vi "FPGA_CounterEncoderSourceConvertionLVSourceTypeToFPGAType.vi"(8 "error in (no error)":errorcluster, 11 "DigitalSource":T1={"DevStatus"={"status"=FALSE, "code"=0, "source"=""}, "AnalogTriggerMode?"=FALSE, "DigitalMode"={"DIO Channel"=enum."DIO 1"}, "AnalogTriggerMode"={"AnalogTriggerIndex"=enum."Trig 0", "OutputType"=enum."InWindow"}}) -> (0 "error out":errorcluster, 3 "FPGASource":T5={"Channel"=2.0, "Module"=0.0, "AnalogTrigger"=FALSE})   [LabVIEW 2017]
uses:
  <vilib>/Rock Robotics/SystemInterfaces/CounterEncoderSourceConvertion/FPGA_CounterEncoderSourceConvertionLVSourceType.ctl
  <vilib>/Rock Robotics/SystemInterfaces/DIO/FPGA_DIODigitalSourceChannel.ctl
  <vilib>/Rock Robotics/SystemInterfaces/AnalogTrigger/FPGA_AnalogTriggerIndex.ctl
  <vilib>/Rock Robotics/SystemInterfaces/AnalogTrigger/FPGA_AnalogTriggerOutType.ctl
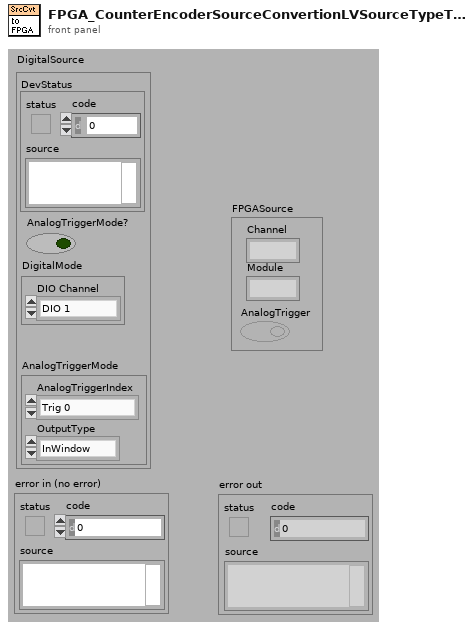
[diagram p1: front panel]
types:
  T1 = typedef "FPGA_CounterEncoderSourceConvertionLVSourceType.ctl" = cluster{"DevStatus":errorcluster, "AnalogTriggerMode?":bool, "DigitalMode":cluster{"DIO Channel":T2}, "AnalogTriggerMode":cluster{"AnalogTriggerIndex":T3, "OutputType":T4}}
  T2 = typedef "FPGA_DIODigitalSourceChannel.ctl" = enum8{"DIO 0", "DIO 1", "DIO 2", "DIO 3", "DIO 4", "DIO 5", "DIO 6", "DIO 7", "DIO 8", "DIO 9", "DIO MXP 0", "DIO MXP 1", "DIO MXP 2", "DIO MXP 3", "DIO MXP 4", "DIO MXP 5", "DIO MXP 6", "DIO MXP 7", "DIO MXP 8", "DIO MXP 9", "DIO MXP 10", "DIO MXP 11", "DIO MXP 12", "DIO MXP 13", "DIO MXP 14", "DIO MXP 15", "Disabled"}
  T3 = typedef "FPGA_AnalogTriggerIndex.ctl" = enum8{"Trig 0", "Trig 1", "Trig 2", "Trig 3", "Trig 4", "Trig 5", "Trig 6", "Trig 7", "Invalid"}
  T4 = typedef "FPGA_AnalogTriggerOutType.ctl" = enum16{"InWindow", "TriggerState", "Rising", "Falling"}
  T5 = cluster{"Channel":fxp<+,4,4>, "Module":fxp<+,1,1>, "AnalogTrigger":bool}
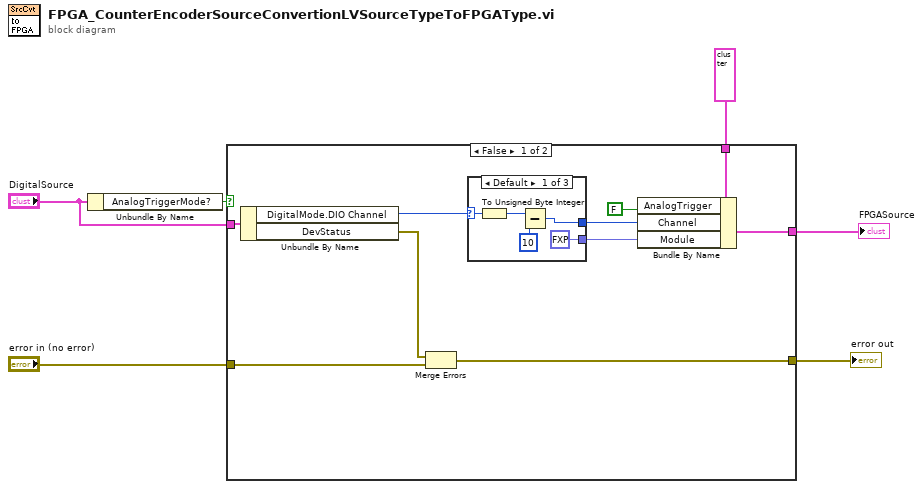
[diagram p0: block diagram]
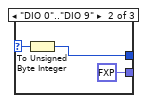
[diagram p2: hidden frame]
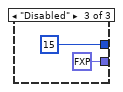
[diagram p3: hidden frame]
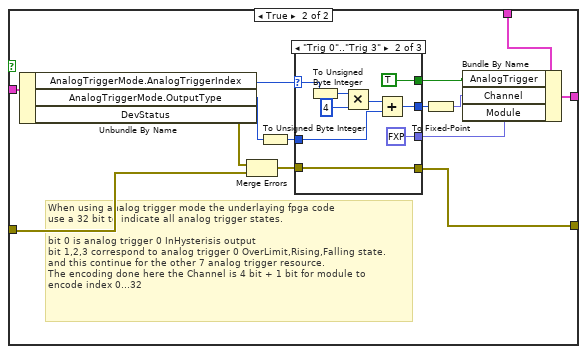
[diagram p4: hidden frame]
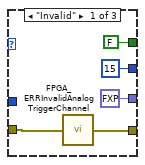
[diagram p5: hidden frame]
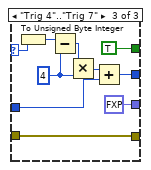
[diagram p6: hidden frame]
diagram:
  n1 = Unbundle By Name("DigitalSource") -> ("AnalogTriggerMode?"=w1:bool)
  n2 = case shown="False" w1 {
    tunnel: "DigitalSource" -> [w16 w38]
    tunnel: [w10 w32] -> w6
    tunnel: T5 {"Channel"=0.0, "Module"=0.0, "AnalogTrigger"=FALSE} ("FPGASource") -> [w15 w40]
    tunnel: [w14 w39] -> w4
    tunnel: "error in (no error)" -> [w12 w29]
    frame False {
      n3 = Unbundle By Name(w16) -> ("DigitalMode.DIO Channel"=w7:T2, "DevStatus"=w11:errorcluster)
      n4 = Merge Errors(w11, w12) -> (w10:errorcluster)
      n5 = case shown="Default" w7 {
        selector: w7 -> [w20 w24 _]
        tunnel: [w19 w22 u8 15 ("unsigned 8bit integer")] -> w9
        tunnel: [fxp<+,1,1> 1.0 ("Module") fxp<+,1,1> 0.0 ("Module") fxp<+,1,1> 0.0 ("Module")] -> w8
        frame Default {
          n6 = To Unsigned Byte Integer(number=w20) -> (unsigned 8bit integer=w17:u8)
          n7 = Subtract(x=w17, y=u8 10) -> (x-y=w19:u8)
        }
        frame "DIO 0".."DIO 9" {
          n8 = To Unsigned Byte Integer(number=w24) -> (unsigned 8bit integer=w22:u8)
        }
        frame "Disabled" {
        }
      }
      n9 = Bundle By Name(cluster=w15, "AnalogTrigger"=FALSE, "Channel"=w9, "Module"=w8) -> (w14:T5)
    }
    frame True {
      # "When using analog trigger mode the underlaying fpga code\nuse a 32 bit to indicate all analog trigger states.\n\nbit 0 is analog trigger 0 InHysterisis output\nbit 1,2,3 correspond to analog trigger 0 OverLimit,Rising,Falling state.\nand this continue for the other 7 analog trigger resource.\nThe encoding done here the Channel is 4 bit + 1 bit for module to \nencode index 0...32"
      n10 = Unbundle By Name(w38) -> ("AnalogTriggerMode.AnalogTriggerIndex"=w31:T3, "AnalogTriggerMode.OutputType"=w37:T4, "DevStatus"=w30:errorcluster)
      n11 = Merge Errors(w30, w29) -> (w28:errorcluster)
      n12 = To Unsigned Byte Integer(number=w37) -> (unsigned 8bit integer=w36:u8)
      n13 = case shown="\"Trig 0\"..\"Trig 3\"" w31 {
        selector: w31 -> [_ w54 w64]
        tunnel: w36 -> [_ w50 w62]
        tunnel: [u8 15 w49 w61] -> w35
        tunnel: [fxp<+,1,1> 0.0 ("Module") fxp<+,1,1> 0.0 ("Module") fxp<+,1,1> 1.0 ("Module")] -> w34
        tunnel: [w42 w47 w56] -> w32
        tunnel: w28 -> [w43 w47 w56]
        tunnel: [FALSE ("AnalogTrigger") TRUE ("AnalogTrigger") TRUE ("AnalogTrigger")] -> w27
        frame "Invalid" {
          n14 = call <vilib>:"FPGA_ERRInvalidAnalogTriggerChannel.vi"("error in (no error)"=w43) -> ("error out"=w42:errorcluster)
        }
        frame "Trig 0".."Trig 3" {
          n15 = To Unsigned Byte Integer(number=w54) -> (unsigned 8bit integer=w53:u8)
          n16 = Multiply(x=w53, y=u8 4) -> (x*y=w51:u8)
          n17 = Add(x=w51, y=w50) -> (x+y=w49:u8)
        }
        frame "Trig 4".."Trig 7" {
          w59 = u8 4 ("y")
          n18 = To Unsigned Byte Integer(number=w64) -> (unsigned 8bit integer=w60:u8)
          n19 = Subtract(x=w60, y=w59) -> (x-y=w58:u8)
          n20 = Multiply(x=w58, y=w59) -> (x*y=w63:u8)
          n21 = Add(x=w63, y=w62) -> (x+y=w61:u8)
        }
      }
      n22 = To Fixed-Point(number=w35) -> (fixed-point=w33:fxp<+,4,4>)  [unwired: 1 out]
      n23 = Bundle By Name(cluster=w40, "AnalogTrigger"=w27, "Channel"=w33, "Module"=w34) -> (w39:T5)
    }
  }
  "FPGASource" <- w4
  "error out" <- w6
